vi "Additional VI Scripting Type.vi"(8 "error in (no error)":errorcluster, 10 "VI Refnum":refnum<vi>, 11 "Scaffold Project Refs":T1) -> (0 "error out":errorcluster)   [LabVIEW 2018, in "LVClassByRef.lvlib"]
uses:
  <resource>/Framework/Providers/LVClassByRef/LVClassByRef.lvlib
  <resource>/Framework/Providers/LVClassByRef/Scaffold Project Refs.ctl
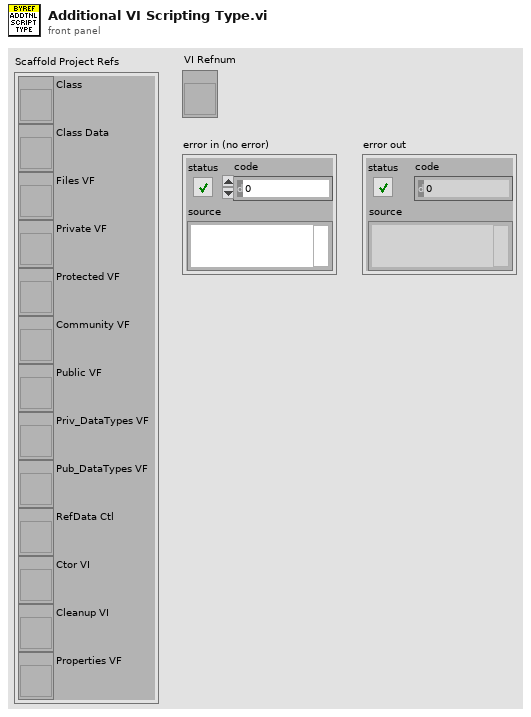
[diagram p1: front panel]
types:
  T1 = typedef "LVClassByRef.lvlib/Scaffold Project Refs.ctl" = cluster{"Class":refnum<vi>, "Class Data":refnum<vi>, "Files VF":refnum<vi>, "Private VF":refnum<vi>, "Protected VF":refnum<vi>, "Community VF":refnum<vi>, "Public VF":refnum<vi>, "Priv_DataTypes VF":refnum<vi>, "Pub_DataTypes VF":refnum<vi>, "RefData Ctl":refnum<vi>, "Ctor VI":refnum<vi>, "Cleanup VI":refnum<vi>, "Properties VF":refnum<vi>}
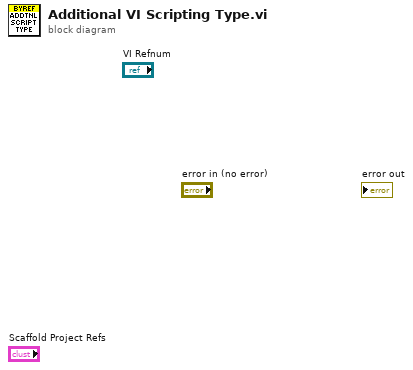
[diagram p0: block diagram]
diagram:
